vi "Calculate Center.vi"(8 "Type of Assembly Tray":i32, 9 "Syringe Coordinates":dbl[](array[numeric]), 10 "Relative Coordinates":dbl[][](array[numeric]), 11 "Fiducial Measurements":dbl[][](array[numeric])) -> (3 "XYZTheta Centers":dbl[][](array[numeric]))   [LabVIEW 2016, in "Baseplate Tray.lvclass"]
uses:
  Baseplate Tray.lvclass
  <vilib>/Analysis/coordinate.llb/2D Cartesian Coordinate Rotation (Scalar).vi
  <vilib>/Analysis/NI_AALPro.lvlib
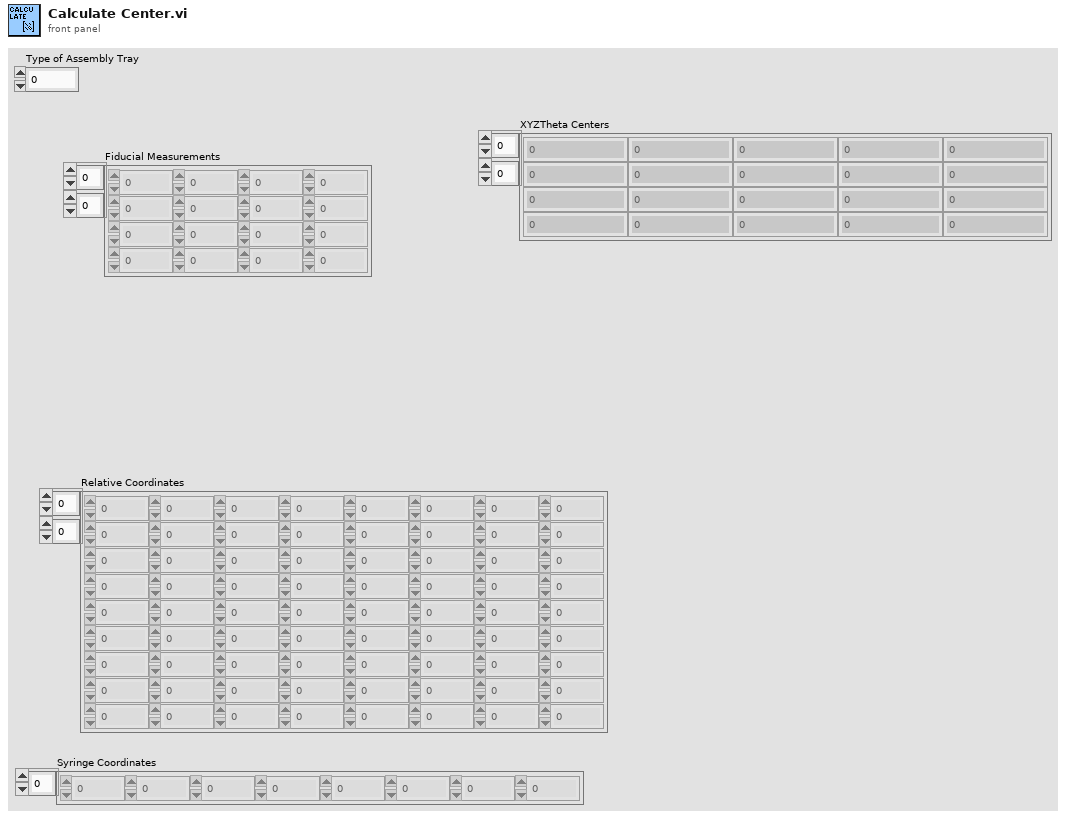
[diagram p1: front panel]
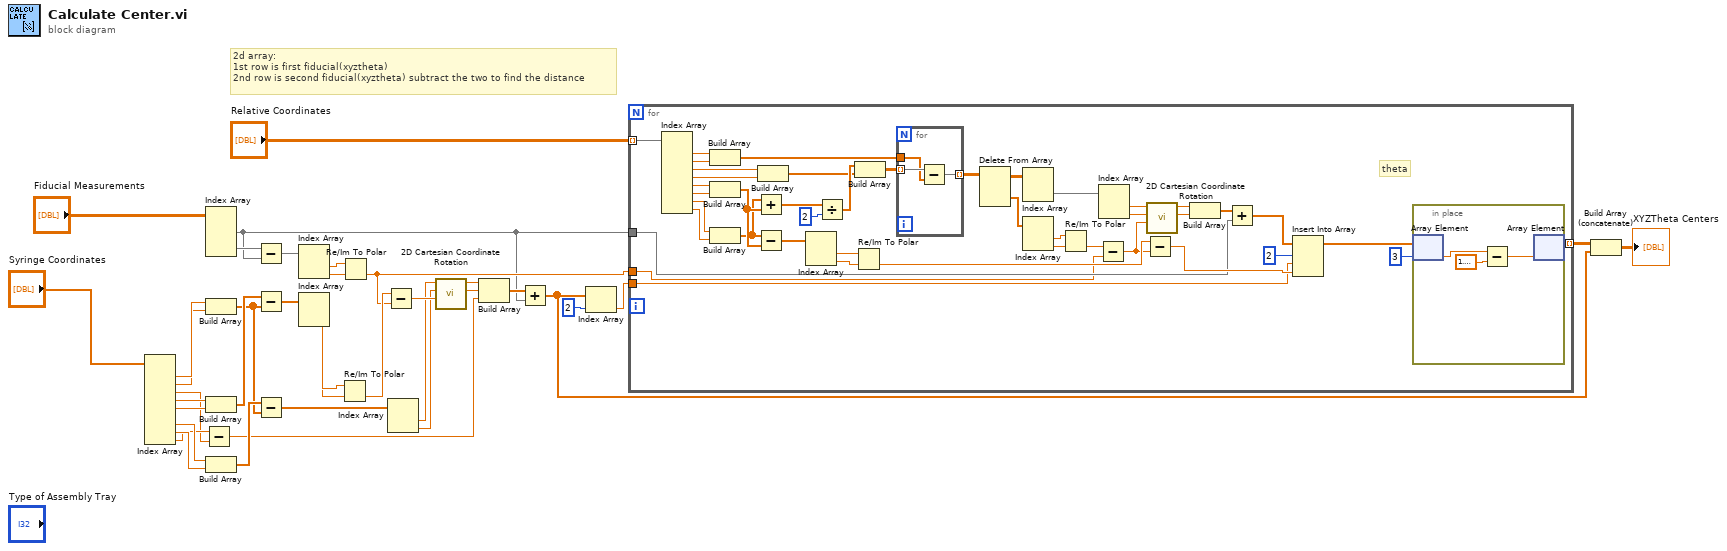
[diagram p0: block diagram]
diagram:
  # "2d array:\n1st row is first fiducial(xyztheta)\n2nd row is second fiducial(xyztheta) subtract the two to find the distance"
  n1 = Index Array(array="Syringe Coordinates") -> (element #1=w31:dbl, element #2=w30:dbl, element #3=w12:dbl, element #4=w28:dbl, element #5=w27:dbl, element #7=w15:dbl, element #8=w14:dbl, element #9=w13:dbl)  [unwired: 9 in, 1 out]
  n2 = Subtract(x=w13, y=w12) -> (x-y=w4:dbl)
  n3 = Index Array(array="Fiducial Measurements") -> (element #1=w3:dbl[], element #2=w34:dbl[])  [unwired: 4 in]
  n4 = Build Array(w31, w30) -> (w19:dbl[])
  n5 = Build Array(w28, w27) -> (w29:dbl[])
  n6 = Build Array(w15, w14) -> (w20:dbl[])
  n7 = Subtract(x=w34, y=w3) -> (x-y=w7:dbl[])
  n8 = Subtract(x=w29, y=w19) -> (x-y=w26:dbl[])
  n9 = Subtract(x=w20, y=w19) -> (x-y=w18:dbl[])
  n10 = Index Array(array=w7) -> (element #1=w35:dbl, element #2=w36:dbl)  [unwired: 2 in]
  n11 = Index Array(array=w26) -> (element #1=w25:dbl, element #2=w24:dbl)  [unwired: 2 in]
  n12 = Re/Im To Polar(2:w24, 3:w25) -> (0:w23:dbl)  [unwired: 1 out]
  n13 = Re/Im To Polar(2:w36, 3:w35) -> (0:w22:dbl)  [unwired: 1 out]
  n14 = Subtract(x=w23, y=w22) -> (x-y=w21:dbl)
  n15 = Index Array(array=w18) -> (element #1=w17:dbl, element #2=w16:dbl)  [unwired: 2 in]
  n16 = call-poly <vilib>:"2D Cartesian Coordinate Rotation.vi"("theta"=w21, "y"=w16, "x"=w17) -> ("y out"=w10:dbl, "x out"=w11:dbl)  [unwired: 6 in, 1 out]
  n17 = Build Array(w11, w10, w4) -> (w8:dbl[])
  n18 = Add(x=w8, y=w3) -> (x+y=w2:dbl[])
  n19 = Index Array(array=w2, index=2) -> (element=w5:dbl)
  n20 = for {
    tunnel: "Relative Coordinates" -> [w44] mode=indexing
    tunnel: w3 -> [w43]
    tunnel: w22 -> [w42]
    tunnel: w5 -> [w41]
    tunnel: [w38] -> w1 mode=indexing
    # "theta"
    n21 = Index Array(array=w44) -> (element #1=w80:dbl, element #2=w79:dbl, element #3=w78:dbl, element #4=w77:dbl, element #5=w76:dbl, element #6=w75:dbl, element #7=w73:dbl, element #8=w74:dbl)  [unwired: 8 in]
    n22 = Build Array(w80, w79) -> (w69:dbl[])
    n23 = Build Array(w76, w75) -> (w52:dbl[])
    n24 = Build Array(w73, w74) -> (w51:dbl[])
    n25 = Add(x=w51, y=w52) -> (x+y=w71:dbl[])
    n26 = Subtract(x=w51, y=w52) -> (x-y=w50:dbl[])
    n27 = Build Array(w78, w77) -> (w54:dbl[])
    n28 = Index Array(array=w50) -> (element #1=w49:dbl, element #2=w48:dbl)  [unwired: 2 in]
    n29 = Divide(x=w71, y=2) -> (x/y=w55:dbl[])
    n30 = Re/Im To Polar(2:w48, 3:w49) -> (0:w47:dbl)  [unwired: 1 out]
    n31 = Build Array(w55, w54) -> (w70:dbl[][])
    n32 = for {
      tunnel: w70 -> [w86] mode=indexing
      tunnel: w69 -> [w85]
      tunnel: [w84] -> w68 mode=indexing
      n33 = Subtract(x=w86, y=w85) -> (x-y=w84:dbl[])
    }
    n34 = Delete From Array(array=w68) -> (deleted portion=w67:dbl[], array with subset deleted=w64:dbl[][])  [unwired: 3 in]
    n35 = Index Array(array=w64) -> (element=w63:dbl[])  [unwired: 2 in]
    n36 = Index Array(array=w67) -> (element #1=w66:dbl, element #2=w65:dbl)  [unwired: 2 in]
    n37 = Re/Im To Polar(2:w65, 3:w66) -> (0:w53:dbl)  [unwired: 1 out]
    n38 = Subtract(x=w53, y=w42) -> (x-y=w45:dbl)
    n39 = Index Array(array=w63) -> (element #1=w62:dbl, element #2=w61:dbl)  [unwired: 2 in]
    n40 = Subtract(x=w47, y=w45) -> (x-y=w46:dbl)
    n41 = call-poly <vilib>:"2D Cartesian Coordinate Rotation.vi"("theta"=w45, "y"=w61, "x"=w62) -> ("y out"=w58:dbl, "x out"=w59:dbl)  [unwired: 6 in, 1 out]
    n42 = Build Array(w59, w58) -> (w60:dbl[])
    n43 = Add(x=w60, y=w43) -> (x+y=w57:dbl[])
    n44 = Insert Into Array "Insert Into Array"(array=w57, index=2, new element #1=w41, new element #2=w46) -> (w40:dbl[])
    n45 = in-place {
      n46 = in-place-array #1(w40, 3) -> (w83:dbl)
      n47 = Subtract(x=w83, y=1.5707963267948966) -> (x-y=w81:dbl)
      n48 = in-place-array #1(w81) -> (w38:dbl[])  [unwired: 1 out]
    }
  }
  n49 = Build Array (concatenate)(w1, w2) -> (→"XYZTheta Centers":dbl[][])
